vi "Set Revision From Module Information.vi"(8 "error in (no error)":errorcluster, 10 "Module Information":T1, 11 "Routing and Faulting Ref in":T3 format="%.0x") -> (0 "error out":errorcluster, 3 "Routing and Faulting Ref out":T3 format="%.0x")   [LabVIEW 2017, in "Routing and Faulting Scripting.lvlib"]
uses:
  Routing and Faulting Scripting.lvlib
  <vilib>/NI Veristand/Custom Device API/Custom Device Item Ref.ctl
  Types/Module Information.ctl
  Shared/Routing and Faulting Hardware API/Types/Possible Connections for Endpoint.ctl
  <vilib>/NI Veristand/Custom Device API/Custom Device API.lvlib
  Shared/Routing and Faulting Hardware API/Routing and Faulting Hardware API.lvlib
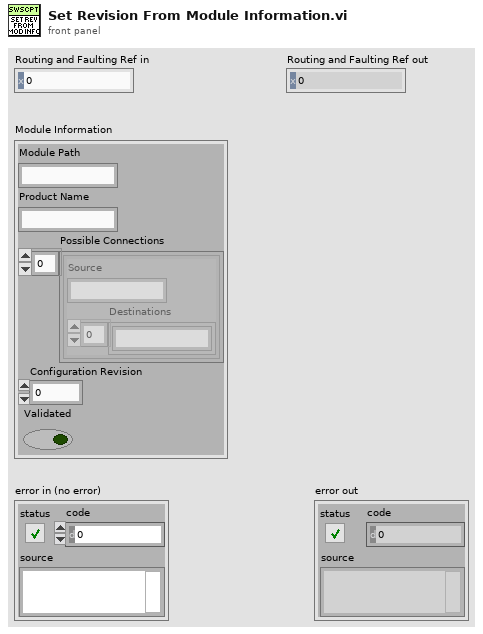
[diagram p1: front panel]
types:
  T1 = typedef "Routing and Faulting Scripting.lvlib/Module Information.ctl" = cluster{"Module Path":string, "Product Name":string, "Possible Connections":T2[], "Configuration Revision":u32, "Validated":bool}
  T2 = typedef "Routing and Faulting Hardware API.lvlib/Possible Connections for Endpoint.ctl" = cluster{"Source":string, "Destinations":string[]}
  T3 = typedef "Custom Device API.lvlib/Custom Device Item Ref.ctl" = u64
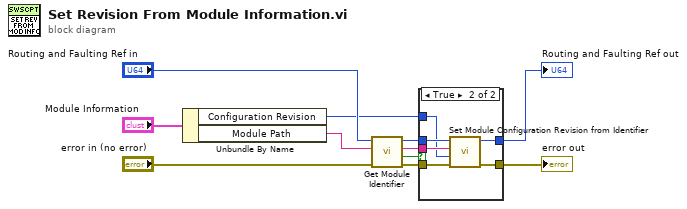
[diagram p0: block diagram]
diagram:
  n1 = Unbundle By Name("Module Information") -> ("Configuration Revision"=w4:u32, "Module Path"=w10:string)
  n2 = call "Get Module Identifier.vi"("error in (no error)"="error in (no error)", "Module path"=w10, "Routing and Faulting Ref in"="Routing and Faulting Ref in") -> ("error out"=w7:errorcluster, "Found?"=w1:bool, "Module identifier"=w5:string, "Routing and Faulting Ref out"=w6:T3)  [unwired: 5 in]
  n3 = case shown="True" w1 {
    tunnel: w7 -> [w12 w19]
    tunnel: w6 -> [w13 w18]
    tunnel: w5 -> [_ w17]
    tunnel: w4 -> [_ w16]
    tunnel: [w12 w15] -> w3
    tunnel: [w13 w14] -> w2
    frame False {
    }
    frame True {
      n4 = call "Set Module Configuration Revision from Identifier.vi"("error in (no error)"=w19, "Revision"=w16, "Module identifier"=w17, "Routing and Faulting Ref in"=w18) -> ("error out"=w15:errorcluster, "Routing and Faulting Ref out"=w14:T3)  [unwired: 6 in]
    }
  }
  "Routing and Faulting Ref out" <- w2
  "error out" <- w3
